vi "CalcRates.vi"(8 "GDT":dbl, 9 "SFDT":dbl, 10 "LT":dbl, 11 "Counts":u32) -> (1 "Cor LT":dbl, 2 "Cor Rate":dbl, 3 "Rate":dbl)   [LabVIEW 2013]
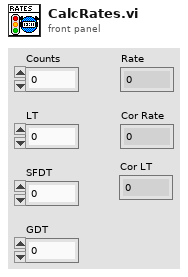
[diagram p1: front panel]
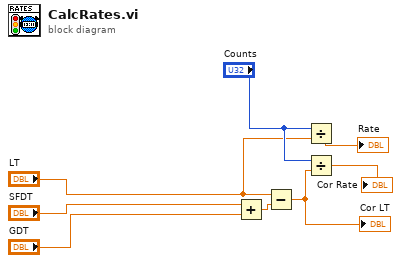
[diagram p0: block diagram]
diagram:
  n1 = Add(x="SFDT", y="GDT") -> (x+y=w3:dbl)
  n2 = Subtract(x="LT", y=w3) -> (x-y=w7:dbl)
  "Cor LT" <- w7
  n3 = Divide(x="Counts", y="LT") -> (x/y=→"Rate":dbl)
  n4 = Divide(x="Counts", y=w7) -> (x/y=→"Cor Rate":dbl)
